vi "Get Available Interactions.vi"(8 "error in":errorcluster, 11 "reference":refnum<k24>) -> (0 "error out":errorcluster, 1 "Interaction Ranges":cluster{"From":dbl, "To":dbl}[](array[cluster]), 2 "Interaction Types":string[](array[string]), 3 "reference out":refnum<k24>)   [LabVIEW 2020, in "Topas4.lvlib"]
uses:
  C:/Windows/SysWOW64/Topas4Lib.dll
  Windows/SysWOW64/Topas4Lib.dll
  Topas4.lvlib
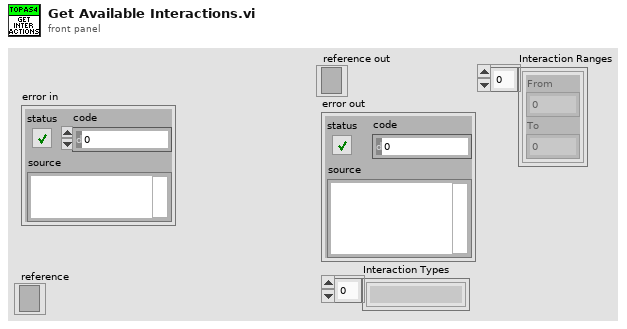
[diagram p1: front panel]
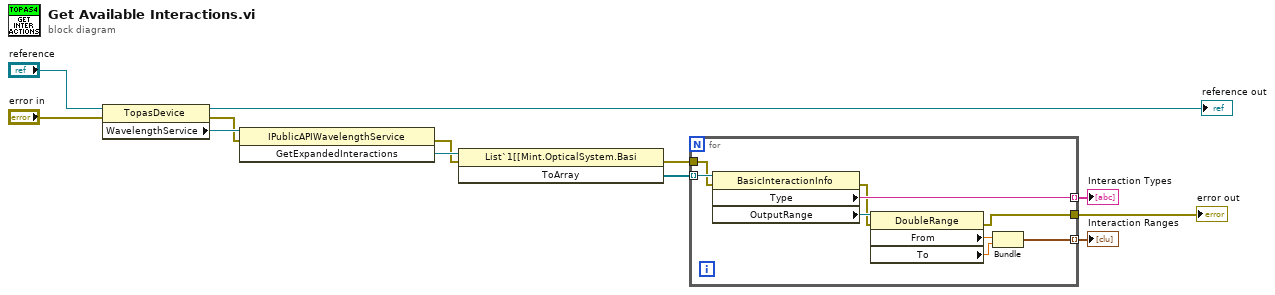
[diagram p0: block diagram]
diagram:
  n1 = property class="TopasDevice"(reference="reference", error in="error in") -> (reference out=→"reference out":refnum<k24>, error out=w8:errorcluster, "WavelengthService"=w9:refnum<k24>)
  n2 = invoke class="IPublicAPIWavelengthService" method="GetExpandedInteractions"(reference=w9, error in=w8) -> (error out=w6:errorcluster, "GetExpandedInteractions"=w7:refnum<k24>)  [unwired: 1 in, 1 out]
  n3 = invoke class="List`1[[Mint.OpticalSystem.Basi" method="ToArray"(reference=w7, error in=w6) -> (error out=w2:errorcluster, "ToArray"=w5:refnum<k24>[])  [unwired: 1 in, 1 out]
  n4 = for {
    tunnel: w5 -> [w21] mode=indexing
    tunnel: [w19] -> w4 mode=indexing
    tunnel: [w16] -> w3 mode=indexing
    tunnel: w2 -> [w15]
    tunnel: [w13] -> w1
    n5 = property class="BasicInteractionInfo"(reference=w21, error in=w15) -> (error out=w14:errorcluster, "Type"=w19:string, "OutputRange"=w20:refnum<k24>)  [unwired: 1 out]
    n6 = property class="DoubleRange"(reference=w20, error in=w14) -> (error out=w13:errorcluster, "From"=w18:dbl, "To"=w17:dbl)  [unwired: 1 out]
    n7 = Bundle("From"=w18, "To"=w17) -> (w16:cluster{"From":dbl, "To":dbl})  [unwired: 1 in]
  }
  "error out" <- w1
  "Interaction Types" <- w4
  "Interaction Ranges" <- w3
